vi "TotalError.vi"(10 "Curren Layer OP":dbl[](array[numeric]), 11 "Target":dbl[](array[numeric])) -> (3 "Numeric":dbl)   [LabVIEW 2014]
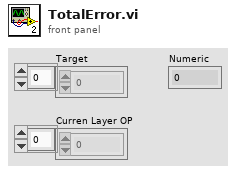
[diagram p1: front panel]
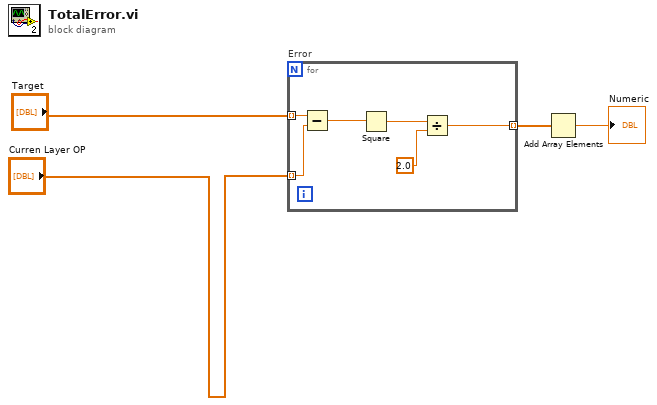
[diagram p0: block diagram]
diagram:
  n1 = for "Error" {
    tunnel: "Target" -> [w7] mode=indexing
    tunnel: "Curren Layer OP" -> [w6] mode=indexing
    tunnel: [w5] -> w1 mode=indexing
    n2 = Subtract(x=w7, y=w6) -> (x-y=w10:dbl)
    n3 = Square(x=w10) -> (x^2=w9:dbl)
    n4 = Divide(x=w9, y=2.0) -> (x/y=w5:dbl)
  }
  n5 = Add Array Elements(numeric array=w1) -> (sum=→"Numeric":dbl)
